vi "element_editor_hydroysis_run.vi"(10 "Break":refnum<vi>) -> ()   [LabVIEW 2019]
uses:
  lib/libSimulationControl/libSimulationControl.lvlib
panel:
  out "spec":path
  # "*******************************************************************\nBiogas Plant Control\n\nAuthor: Paul Zügel\nGCSC-Frankfurt am Main 2020\n\n*******************************************************************"
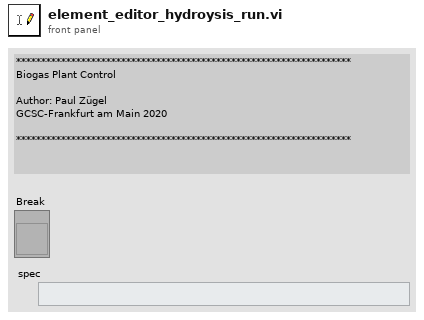
[diagram p1: front panel]
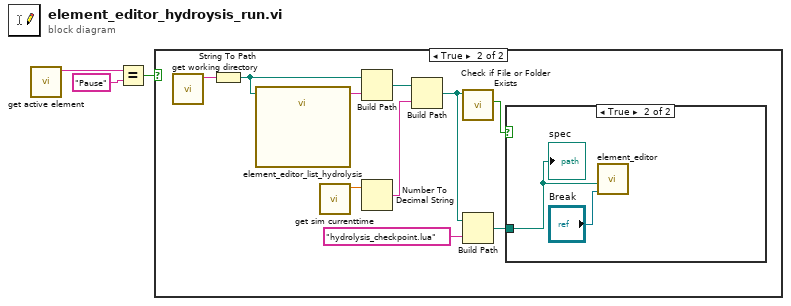
[diagram p0: block diagram]
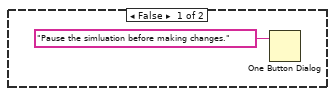
[diagram p2: hidden frame]
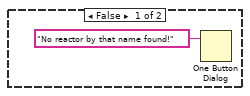
[diagram p3: hidden frame]
diagram:
  n1 = call "get active element.vi"() -> ("active_element"=w3:string)  [unwired: 10 in, 1 out]
  n2 = Equal?(x=w3, y="Pause") -> (x = y?=w1:bool)
  n3 = case shown="True" w1 {
    frame False {
      n4 = One Button Dialog(message="Pause the simluation before making changes.") -> ()  [unwired: 1 in, 1 out]
    }
    frame True {
      n5 = call "get working directory.vi"() -> ("function return"=w14:string)  [unwired: 10 in, 1 out]
      n6 = String To Path(string=w14) -> (path=w5:path)
      n7 = call "element_editor_list_hydrolysis.vi"("path"=w5) -> ("Value"=w13:string)  [unwired: 7 in, 3 out]
      n8 = call "get sim currenttime.vi"() -> ("current_time"=w7:dbl)  [unwired: 10 in, 1 out]
      n9 = Build Path(base path=w5, name or relative path=w13) -> (appended path=w8:path)
      n10 = Number To Decimal String(number=w7) -> (decimal integer string=w9:string)  [unwired: 1 in]
      n11 = Build Path(base path=w8, name or relative path=w9) -> (appended path=w10:path)
      n12 = call <vilib>:"Check if File or Folder Exists.vi"("path"=w10) -> ("file or folder exists?"=w11:bool)  [unwired: 8 in, 2 out]
      n13 = Build Path(base path=w10, name or relative path="hydrolysis_checkpoint.lua") -> (appended path=w12:path)
      n14 = case shown="True" w11 {
        tunnel: w12 -> [_ w16]
        frame False {
          n15 = One Button Dialog(message="No reactor by that name found!") -> ()  [unwired: 1 in, 1 out]
        }
        frame True {
          n16 = call "element_editor.vi"("Break"="Break", "LUA Specification File"=w16) -> ()  [unwired: 5 in, 1 out]
          "spec" <- w16
        }
      }
    }
  }
